vi "GOOP_FirstCall.vi"() -> (3 "First Call?: T/F":bool)   [LabVIEW 2020]
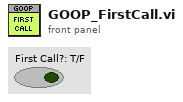
[diagram p1: front panel]
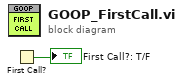
[diagram p0: block diagram]
diagram:
  n1 = First Call?() -> (First Call?: T/F=→"First Call?: T/F":bool)
